vi "Validate.vi"(8 "error in":errorcluster, 10 "Obj Dictionary":refnum<class "Object Dictionary.lvclass">, 11 "Device Profile in":refnum<class "Device Profile.lvclass">) -> (0 "error out":errorcluster, 2 "Missing Objects":T1[](array[typedef]) {"Index" format="%04x"}, 3 "Device Profile out":refnum<class "Device Profile.lvclass">)   [LabVIEW 2020, in "CANopen.lvlib" / "Device Profile.lvclass"]
uses:
  Device Profile.lvclass
  Device Profile.lvclass/Device Profile.ctl
  Object Dictionary/Object Dictionary.lvclass
  Typedefs/OD Entry Spec.ctl
  CANopen.lvlib
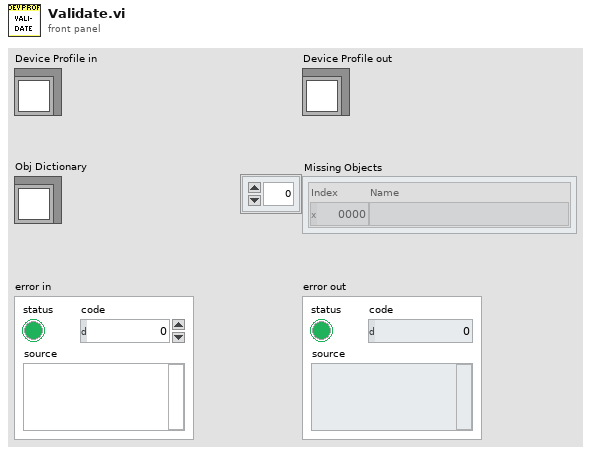
[diagram p1: front panel]
types:
  T1 = typedef "CANopen.lvlib/OD Entry Spec.ctl" = cluster{"Index":u16, "Name":string}
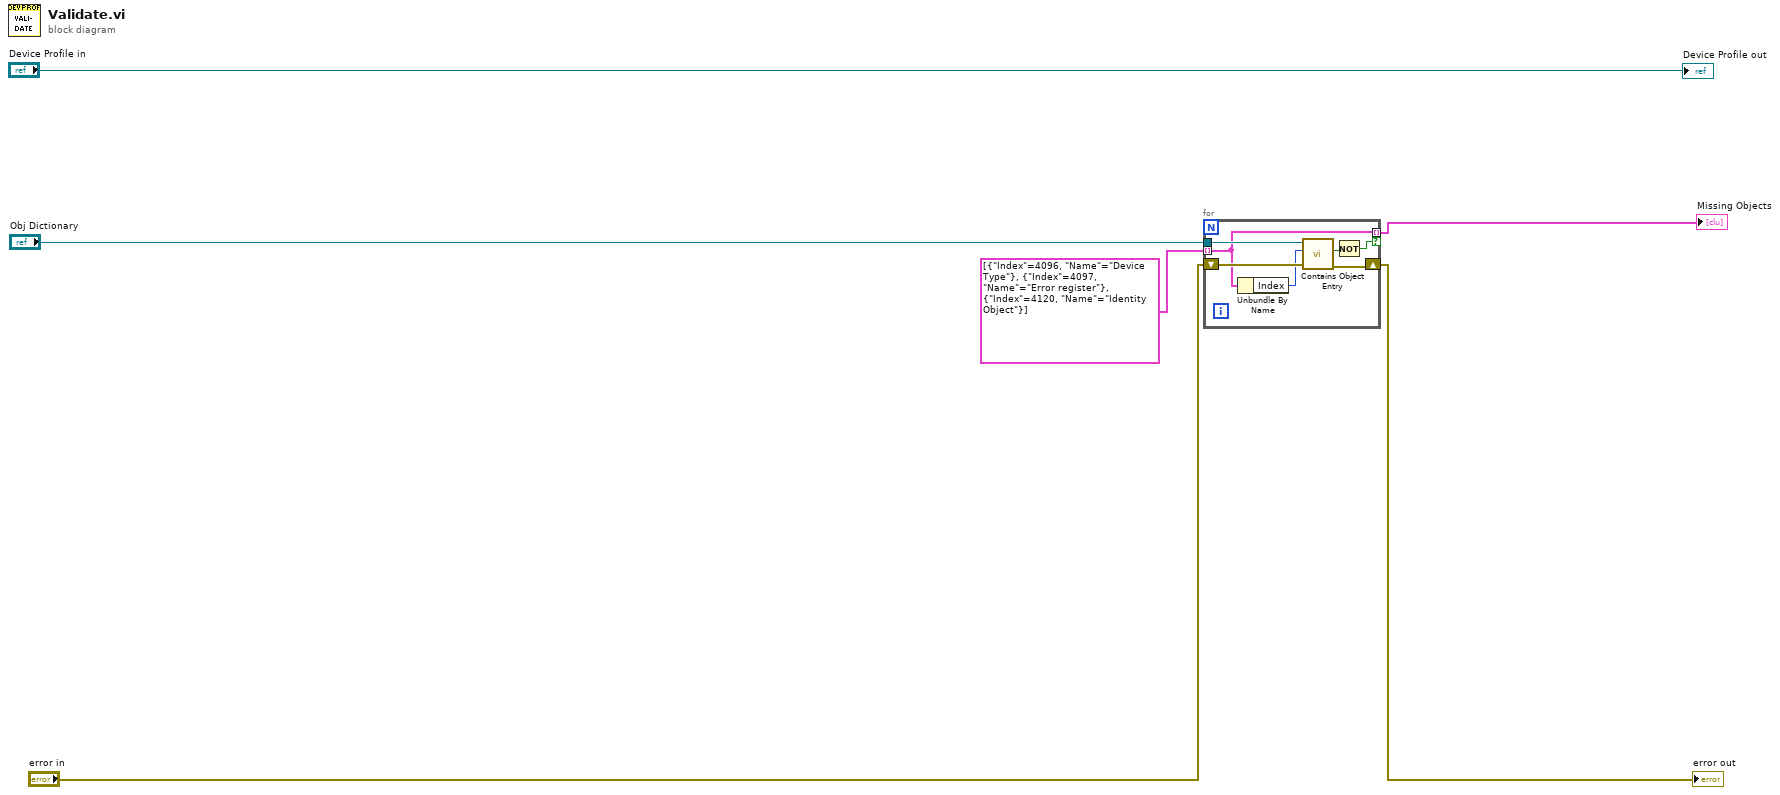
[diagram p0: block diagram]
diagram:
  n1 = for {
    tunnel: "Obj Dictionary" -> [w13]
    tunnel: T1[] [{"Index"=4096, "Name"="Device Type"}, {"Index"=4097, "Name"="Error register"}, {"Index"=4120, "Name"="Identity Object"}] -> [w10] mode=indexing
    shift-right: [w11] -> w4
    shift-left: "error in" -> [w12]
    tunnel: [w10] -> w1 mode=indexing if=w8
    n2 = Unbundle By Name(w10) -> ("Index"=w7:u16)
    n3 = call "Contains Object Entry.vi"("error in"=w12, "OD Index"=w7, "Obj Dict in"=w13) -> ("error out"=w11:errorcluster, "Contains"=w9:bool)  [unwired: 6 in, 1 out]
    n4 = Not(x=w9) -> (.not. x?=w8:bool)
  }
  "error out" <- w4
  "Missing Objects" <- w1
  "Device Profile out" <- "Device Profile in"
